vi "FIR_stage_1.vi"(8 "data valid in":bool, 9 "Q in":fxp<+/-,16,14>[](array[numeric])=[0.0, 0.0, 0.0, 0.0], 10 "I in":fxp<+/-,16,14>[](array[numeric])=[0.0, 0.0, 0.0, 0.0]) -> (0 "data valid out":bool, 1 "Q out":fxp<+/-,20,16>, 2 "I out":fxp<+/-,20,16>)   [LabVIEW 2013]
uses:
  <vilib>/rvi/IPIntegrationNode/IPINode_Utilities/niFpgaIPINodeSimCore.vi
  <vilib>/rvi/FXPMathLib/FxpInterpret/XNode/nifxpmath_Interpret.xnode
  <vilib>/rvi/XilinxIP/XIPIN_XNode/niFpgaXIPIN.xnode
  FIR_stage_1/FIR Compiler/FIR_Compiler_85ED751C02924D88BECD8AD4BEB93A77.dll
  <vilib>/rvi/IPIntegrationNode/IPINode_Xnode/niFpgaIPINode.xnode
  <vilib>/rvi/FXPMathLib/FxpAdd/XNode/nifxpmath_Add.xnode
  FIR_stage_1/FIR Compiler 1 1/FIR_Compiler_1_1_C384D66DF0BE4753A5D47BAB67AE6CF0.dll
  <vilib>/rvi/FXPMathLib/sim/FxpSim.dll
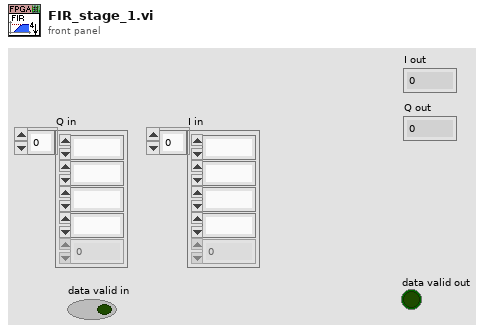
[diagram p1: front panel]
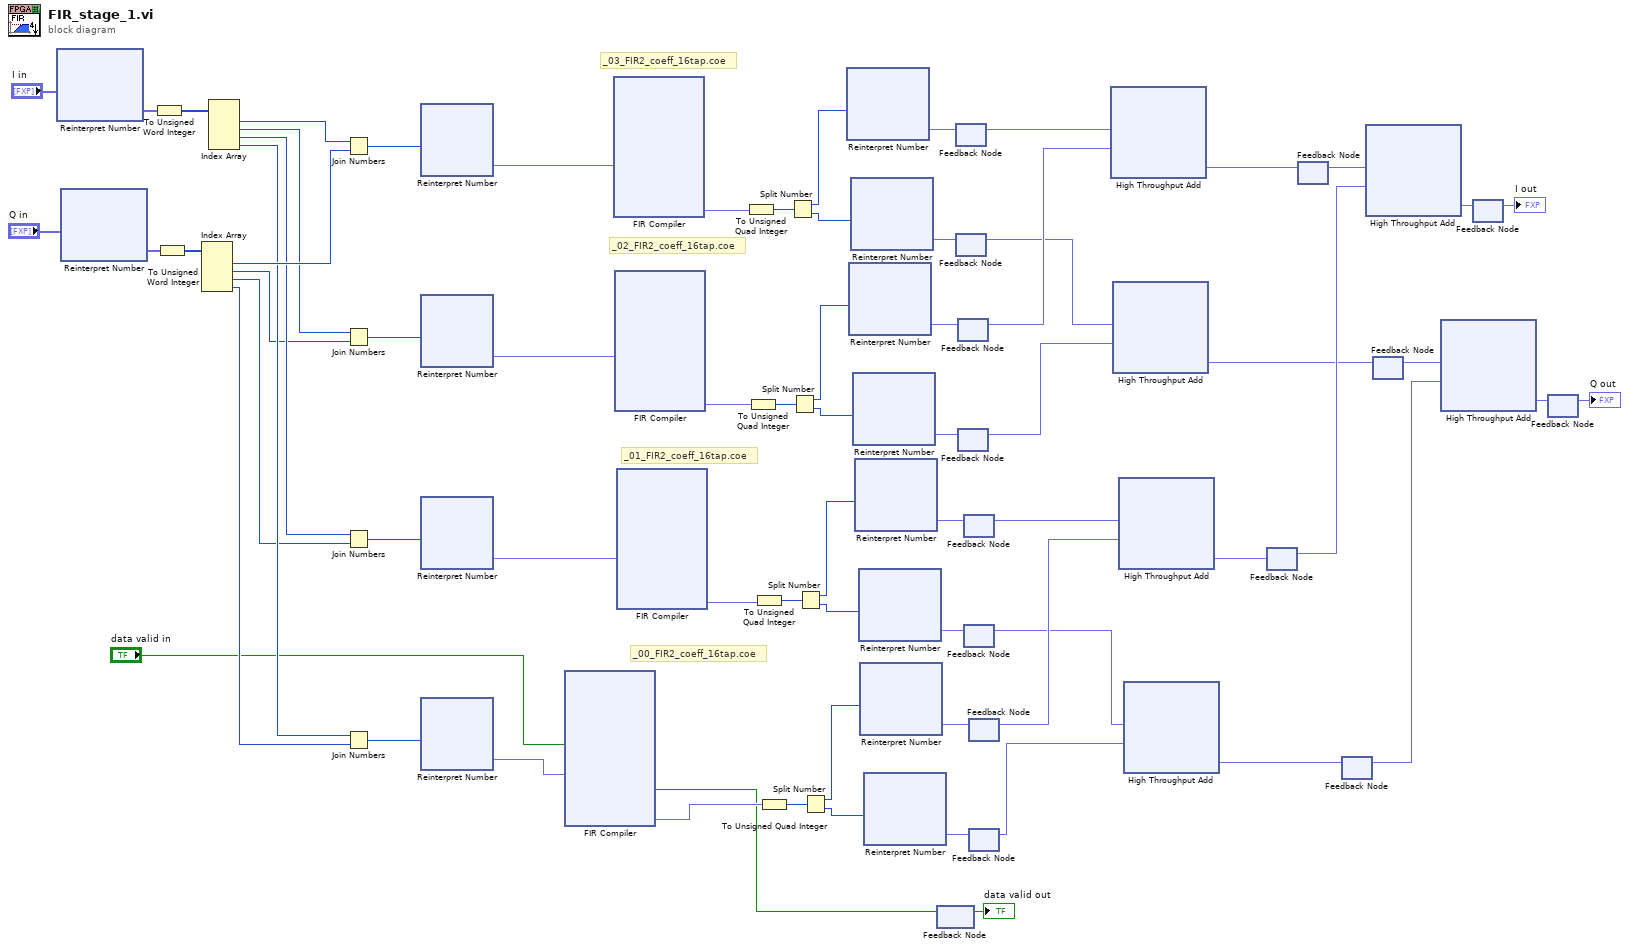
[diagram p0: block diagram]
diagram:
  # "_00_FIR2_coeff_16tap.coe"
  # "_01_FIR2_coeff_16tap.coe"
  # "_02_FIR2_coeff_16tap.coe"
  # "_03_FIR2_coeff_16tap.coe"
  n1 = xnode "Reinterpret Number"("x"="I in") -> ("y"=w5:fxp<+,16,16>[])
  n2 = xnode "Reinterpret Number"("x"="Q in") -> ("y"=w7:fxp<+,16,16>[])
  n3 = To Unsigned Word Integer(number=w5) -> (unsigned 16bit integer=w69:u16[])
  n4 = To Unsigned Word Integer(number=w7) -> (unsigned 16bit integer=w4:u16[])
  n5 = Index Array(array=w4) -> (element #1=w67:u16, element #2=w30:u16, element #3=w29:u16, element #4=w28:u16)  [unwired: 4 in]
  n6 = Index Array(array=w69) -> (element #1=w68:u16, element #2=w33:u16, element #3=w32:u16, element #4=w31:u16)  [unwired: 4 in]
  n7 = Join Numbers(hi=w68, lo=w67) -> ((hi.lo)=w66:u32)
  n8 = Join Numbers(hi=w33, lo=w30) -> ((hi.lo)=w39:u32)
  n9 = Join Numbers(hi=w32, lo=w29) -> ((hi.lo)=w38:u32)
  n10 = Join Numbers(hi=w31, lo=w28) -> ((hi.lo)=w37:u32)
  n11 = xnode "Reinterpret Number"("x"=w66) -> ("y"=w65:fxp<+,32,32>)
  n12 = xnode "Reinterpret Number"("x"=w39) -> ("y"=w36:fxp<+,32,32>)
  n13 = xnode "Reinterpret Number"("x"=w38) -> ("y"=w35:fxp<+,32,32>)
  n14 = xnode "Reinterpret Number"("x"=w37) -> ("y"=w34:fxp<+,32,32>)
  n15 = xnode ("FIR Compiler")("s_axis_data_tvalid"="data valid in", "s_axis_data_tdata"=w34) -> ("m_axis_data_tvalid"=w3:bool, "m_axis_data_tdata"=w42:fxp<+,64,64>)  [unwired: 2 in, 2 out]
  n16 = xnode ("FIR Compiler")("s_axis_data_tdata"=w65) -> ("m_axis_data_tdata"=w64:fxp<+,64,64>)  [unwired: 3 in, 3 out]
  n17 = xnode ("FIR Compiler")("s_axis_data_tdata"=w36) -> ("m_axis_data_tdata"=w40:fxp<+,64,64>)  [unwired: 3 in, 3 out]
  n18 = xnode ("FIR Compiler")("s_axis_data_tdata"=w35) -> ("m_axis_data_tdata"=w41:fxp<+,64,64>)  [unwired: 3 in, 3 out]
  n19 = To Unsigned Quad Integer(1:w64) -> (0:w63:u64)
  n20 = To Unsigned Quad Integer(1:w40) -> (0:w53:u64)
  n21 = To Unsigned Quad Integer(1:w41) -> (0:w52:u64)
  n22 = To Unsigned Quad Integer(1:w42) -> (0:w43:u64)
  n23 = Split Number(x=w63) -> (hi(x)=w61:u32, lo(x)=w59:u32)
  n24 = Split Number(x=w53) -> (hi(x)=w54:u32, lo(x)=w56:u32)
  n25 = Split Number(x=w52) -> (hi(x)=w51:u32, lo(x)=w49:u32)
  n26 = Split Number(x=w43) -> (hi(x)=w44:u32, lo(x)=w46:u32)
  n27 = xnode "Reinterpret Number"("x"=w61) -> ("y"=w60:fxp<+/-,32,14>)
  n28 = xnode "Reinterpret Number"("x"=w54) -> ("y"=w55:fxp<+/-,32,14>)
  n29 = xnode "Reinterpret Number"("x"=w59) -> ("y"=w58:fxp<+/-,32,14>)
  n30 = xnode "Reinterpret Number"("x"=w56) -> ("y"=w57:fxp<+/-,32,14>)
  n31 = xnode "Reinterpret Number"("x"=w51) -> ("y"=w50:fxp<+/-,32,14>)
  n32 = xnode "Reinterpret Number"("x"=w49) -> ("y"=w48:fxp<+/-,32,14>)
  n33 = xnode "Reinterpret Number"("x"=w44) -> ("y"=w45:fxp<+/-,32,14>)
  n34 = xnode "Reinterpret Number"("x"=w46) -> ("y"=w47:fxp<+/-,32,14>)
  n35 = feedback #1() -> (→"data valid out":bool)  [unwired: 1 in]
  n36 = feedback-in #1(w3) -> ()
  n37 = feedback #2() -> (w62:fxp<+/-,32,14>)  [unwired: 1 in]
  n38 = feedback-in #2(w60) -> ()
  n39 = feedback #3() -> (w22:fxp<+/-,32,14>)  [unwired: 1 in]
  n40 = feedback-in #3(w58) -> ()
  n41 = feedback #4() -> (w27:fxp<+/-,32,14>)  [unwired: 1 in]
  n42 = feedback-in #4(w55) -> ()
  n43 = feedback #5() -> (w21:fxp<+/-,32,14>)  [unwired: 1 in]
  n44 = feedback-in #5(w57) -> ()
  n45 = feedback #6() -> (w26:fxp<+/-,32,14>)  [unwired: 1 in]
  n46 = feedback-in #6(w50) -> ()
  n47 = feedback #7() -> (w23:fxp<+/-,32,14>)  [unwired: 1 in]
  n48 = feedback-in #7(w48) -> ()
  n49 = feedback #8() -> (w25:fxp<+/-,32,14>)  [unwired: 1 in]
  n50 = feedback-in #8(w45) -> ()
  n51 = feedback #9() -> (w24:fxp<+/-,32,14>)  [unwired: 1 in]
  n52 = feedback-in #9(w47) -> ()
  n53 = xnode "High Throughput Add"("x"=w62, "y"=w27) -> ("x+y"=w16:fxp<+/-,19,15>)
  n54 = xnode "High Throughput Add"("x"=w22, "y"=w21) -> ("x+y"=w10:fxp<+/-,19,15>)
  n55 = xnode "High Throughput Add"("x"=w26, "y"=w25) -> ("x+y"=w15:fxp<+/-,19,15>)
  n56 = xnode "High Throughput Add"("x"=w23, "y"=w24) -> ("x+y"=w9:fxp<+/-,19,15>)
  n57 = feedback #10() -> (w20:fxp<+/-,19,15>)  [unwired: 1 in]
  n58 = feedback-in #10(w15) -> ()
  n59 = feedback #11() -> (w19:fxp<+/-,19,15>)  [unwired: 1 in]
  n60 = feedback-in #11(w16) -> ()
  n61 = feedback #12() -> (w11:fxp<+/-,19,15>)  [unwired: 1 in]
  n62 = feedback-in #12(w9) -> ()
  n63 = xnode "High Throughput Add"("x"=w19, "y"=w20) -> ("x+y"=w17:fxp<+/-,20,16>)
  n64 = feedback #13() -> (w12:fxp<+/-,19,15>)  [unwired: 1 in]
  n65 = feedback-in #13(w10) -> ()
  n66 = xnode "High Throughput Add"("x"=w12, "y"=w11) -> ("x+y"=w14:fxp<+/-,20,16>)
  n67 = feedback #14() -> (→"I out":fxp<+/-,20,16>)  [unwired: 1 in]
  n68 = feedback-in #14(w17) -> ()
  n69 = feedback #15() -> (→"Q out":fxp<+/-,20,16>)  [unwired: 1 in]
  n70 = feedback-in #15(w14) -> ()
